vi "CheckForWin.vi"(8 "error in (no error)":errorcluster, 11 "Pong in":refnum<class "Pong.lvclass">) -> (0 "error out":errorcluster, 3 "Pong out":refnum<class "Pong.lvclass">)   [LabVIEW 2019, in "RT_Game.lvlib" / "Pong.lvclass"]
uses:
  Pong.lvclass
  C:/Users/FreshBob/Dropbox/VIs/myRIO_GameConsole/RT/RT_Game/Game/Game.lvclass
  Game/Coordinate.ctl
  PongBall/PongBall.lvclass
  C:/Users/FreshBob/Dropbox/VIs/myRIO_GameConsole/RT/RT_Game/GameObject/GameObject.lvclass
  C:/Users/FreshBob/Dropbox/VIs/myRIO_GameConsole/RT/RT_Game/RT_Sprite/RT_Sprite.lvclass
  Game/Game.lvclass/Game.ctl
  GameObject/GameObject.lvclass/GameObject.ctl
  Pong.lvclass/Pong.ctl
  Winners.ctl
  Game/Read Sprite3.vi
  GameObject/Read position.vi
  GameObject/Read size.vi
  Game/Write Sprite3.vi
  RT_Sprite/RT_Sprite.lvclass
  Game/Game.lvclass
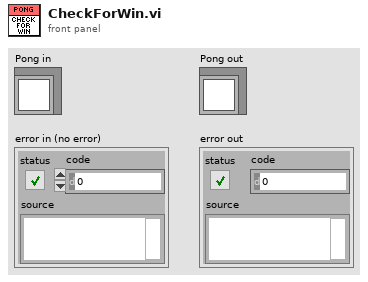
[diagram p1: front panel]
types:
  T1 = typedef "RT_Game.lvlib/Game.lvclass/Coordinate.ctl" = cluster{"x":dbl, "y":dbl}
  T2 = typedef "RT_Game.lvlib/Pong.lvclass/Winners.ctl" = enum16{"None", "Player1", "Player2"}
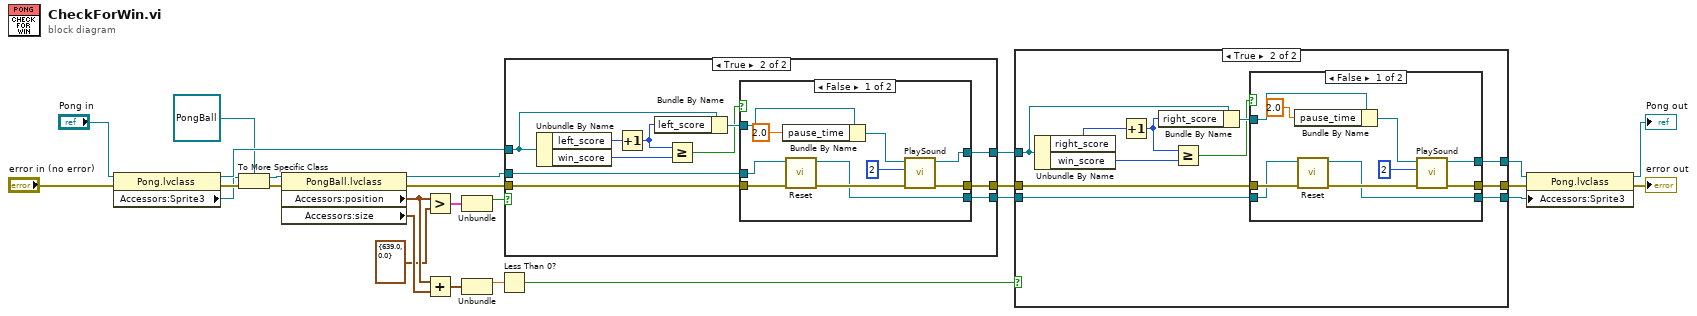
[diagram p0: block diagram]
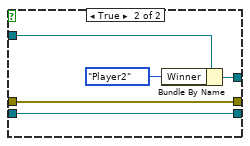
[diagram p3: hidden frame]
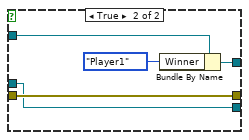
[diagram p5: hidden frame]
diagram:
  n1 = property class="Pong.lvclass"(reference="Pong in", error in="error in (no error)") -> (reference out=w11:refnum<class "Pong.lvclass">, error out=w13:errorcluster, "Accessors:Sprite3"=w8:refnum<class "RT_Sprite.lvclass">)
  n2 = To More Specific Class(target class=refnum<class "PongBall.lvclass"> refnum ("RT_Game.lvlib:PongBall.lvclass"), reference=w8, error in=w13) -> (specific class reference=w7:refnum<class "PongBall.lvclass">, error out=w10:errorcluster)
  n3 = property class="PongBall.lvclass"(reference=w7, error in=w10) -> (reference out=w6:refnum<class "PongBall.lvclass">, error out=w22:errorcluster, "Accessors:position"=w17:T1, "Accessors:size"=w21:T1)
  n4 = Greater?(x=w17, y=T1 {"x"=639.0, "y"=0.0}) -> (0:w15:cluster{"x":bool, "y":bool})
  n5 = Add(x=w17, y=w21) -> (x+y=w20:T1)
  n6 = Unbundle(w15) -> ("x"=w14:bool)  [unwired: 1 out]
  n7 = Unbundle(w20) -> ("x"=w19:dbl)  [unwired: 1 out]
  n8 = Less Than 0?(x=w19) -> (x < 0?=w18:bool)
  n9 = case shown="True" w14 {
    tunnel: [w29 w36] -> w26
    tunnel: w11 -> [w29 w39]
    tunnel: w22 -> [w28 w33]
    tunnel: [w28 w32] -> w25
    tunnel: w6 -> [w27 w31]
    tunnel: [w27 w30] -> w2
    frame False {
    }
    frame True {
      n10 = Unbundle By Name(w39) -> ("left_score"=w38:i16, "win_score"=w34:i16)
      n11 = Increment(x=w38) -> (x+1=w37:i16)
      n12 = Bundle By Name(cluster=w39, "left_score"=w37) -> (w40:refnum<class "Pong.lvclass">)
      n13 = Greater Or Equal?(x=w37, y=w34) -> (x >= y?=w35:bool)
      n14 = case shown="False" w35 {
        tunnel: w40 -> [w50 w55]
        tunnel: [w45 w54] -> w36
        tunnel: w33 -> [w49 w52]
        tunnel: [w46 w52] -> w32
        tunnel: w31 -> [w42 w51]
        tunnel: [w41 w51] -> w30
        frame False {
          n15 = Bundle By Name(cluster=w50, "pause_time"=2.0) -> (w43:refnum<class "Pong.lvclass">)
          n16 = call "Reset.vi"("error in (no error)"=w49, "PongBall in"=w42) -> ("error out"=w47:errorcluster, "PongBall out"=w41:refnum<class "PongBall.lvclass">)  [unwired: 8 in]
          n17 = call "PlaySound.vi"("error in (no error)"=w47, "Index"=i16 2, "Game in"=w43) -> ("error out"=w46:errorcluster, "Game out"=w45:refnum<class "Pong.lvclass">)  [unwired: 7 in]
        }
        frame True {
          n18 = Bundle By Name(cluster=w55, "Winner"=Winners."Player1") -> (w54:refnum<class "Pong.lvclass">)
        }
      }
    }
  }
  n19 = case shown="True" w18 {
    tunnel: [w58 w65] -> w4
    tunnel: w26 -> [w58 w68]
    tunnel: w25 -> [w57 w62]
    tunnel: [w57 w61] -> w24
    tunnel: w2 -> [w56 w60]
    tunnel: [w56 w59] -> w1
    frame False {
    }
    frame True {
      n20 = Unbundle By Name(w68) -> ("right_score"=w67:i16, "win_score"=w63:i16)
      n21 = Increment(x=w67) -> (x+1=w66:i16)
      n22 = Bundle By Name(cluster=w68, "right_score"=w66) -> (w69:refnum<class "Pong.lvclass">)
      n23 = Greater Or Equal?(x=w66, y=w63) -> (x >= y?=w64:bool)
      n24 = case shown="False" w64 {
        tunnel: w69 -> [w78 w84]
        tunnel: [w73 w83] -> w65
        tunnel: w62 -> [w77 w81]
        tunnel: [w75 w81] -> w61
        tunnel: w60 -> [w71 w80]
        tunnel: [w70 w80] -> w59
        frame False {
          n25 = Bundle By Name(cluster=w78, "pause_time"=2.0) -> (w74:refnum<class "Pong.lvclass">)
          n26 = call "Reset.vi"("error in (no error)"=w77, "PongBall in"=w71) -> ("error out"=w76:errorcluster, "PongBall out"=w70:refnum<class "PongBall.lvclass">)  [unwired: 8 in]
          n27 = call "PlaySound.vi"("error in (no error)"=w76, "Index"=i16 2, "Game in"=w74) -> ("error out"=w75:errorcluster, "Game out"=w73:refnum<class "Pong.lvclass">)  [unwired: 7 in]
        }
        frame True {
          n28 = Bundle By Name(cluster=w84, "Winner"=Winners."Player2") -> (w83:refnum<class "Pong.lvclass">)
        }
      }
    }
  }
  n29 = property class="Pong.lvclass"(reference=w4, error in=w24, "Accessors:Sprite3"=w1) -> (reference out=→"Pong out":refnum<class "Pong.lvclass">, error out=→"error out":errorcluster)
